vi "Write AppOutput.vi"(8 "error in (no error)":errorcluster, 10 "RingdownOutput":T1, 11 "VisualizeAppRingdown in":refnum<class "VisualizeAppERA.lvclass">) -> (0 "error out":errorcluster, 3 "VisualizeAppRingdown out":refnum<class "VisualizeAppERA.lvclass">)   [LabVIEW 2017, in "Visualization.lvlib" / "VisualizeAppERA.lvclass"]
uses:
  VisualizeAppERA.lvclass
  Modules/AppPlugins/EraPlugin/PublicAPI/TypeDef/ERAOutput.ctl
  VisualizeAppERA.lvclass/VisualizeAppERA.ctl
  Modules/AppPlugins/EraPlugin/EraPlugin.lvclass
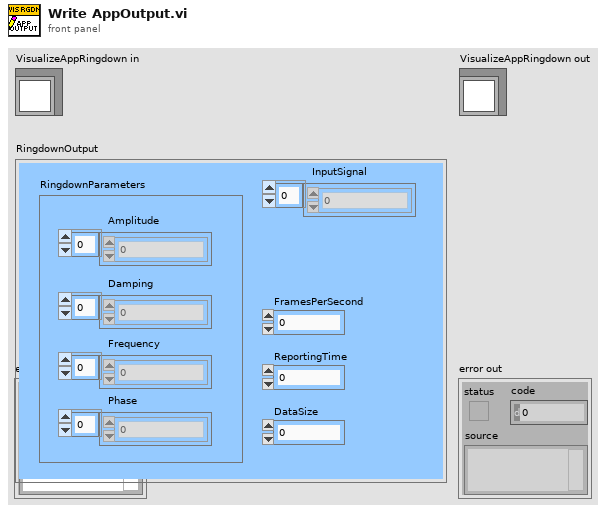
[diagram p1: front panel]
types:
  T1 = typedef "AppPlugins.lvlib/ERAPlugin.lvclass/ERAOutput.ctl" = cluster{"FramesPerSecond":dbl, "RingdownParameters":cluster{"Amplitude":dbl[], "Damping":dbl[], "Frequency":dbl[], "Phase":dbl[]}, "ReportingTime":dbl, "DataSize":u32, "InputSignal":dbl[]}
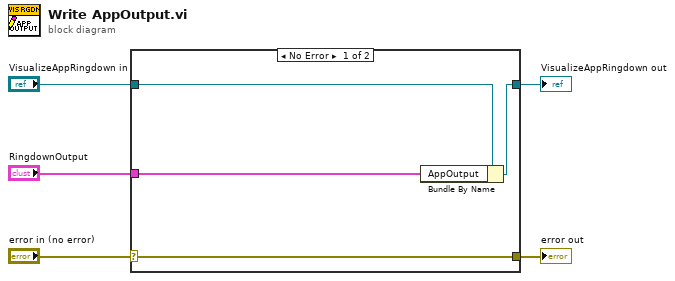
[diagram p0: block diagram]
diagram:
  n1 = case shown="No Error" "error in (no error)" {
    selector: "error in (no error)" -> [w9 w10]
    tunnel: [w9 w10] -> w4
    tunnel: [w7 w11] -> w2
    tunnel: "VisualizeAppRingdown in" -> [w8 w11]
    tunnel: "RingdownOutput" -> [w6 _]
    frame No Error {
      n2 = Bundle By Name(cluster=w8, "AppOutput"=w6) -> (w7:refnum<class "VisualizeAppERA.lvclass">)
    }
    frame Error {
    }
  }
  "error out" <- w4
  "VisualizeAppRingdown out" <- w2
